vi "Main.vi"(8 "error in":errorcluster, 11 "Settings View in":refnum<class "Settings View.lvclass">) -> (0 "error out":errorcluster, 3 "Settings View out":refnum<class "Settings View.lvclass">)   [LabVIEW 2018, in "Settings View.lvclass"]
doc: "The Queued Message Handler of a Worker."
uses:
  Settings View.lvclass
  D:/Program Files (x86)/National Instruments/LabVIEW 2018/vi.lib/addons/_Workers/Library/Classes/Worker/Worker.lvclass
  Initialization Data.ctl
  Settings View.lvclass/Settings View.ctl
  <vilib>/addons/_Workers/Library/Classes/Worker/Worker.lvclass
panel:
  in  "TempSensor":refnum<visa-resource-name>
  in  "PS10":refnum<visa-resource-name>
  in  "PS9":refnum<visa-resource-name>
  in  "PS8":refnum<visa-resource-name>
  in  "PS7":refnum<visa-resource-name>
  in  "PS6":refnum<visa-resource-name>
  in  "PS5":refnum<visa-resource-name>
  in  "PS4":refnum<visa-resource-name>
  in  "PS3":refnum<visa-resource-name>
  in  "PS2":refnum<visa-resource-name>
  in  "PS1":refnum<visa-resource-name>
  in  "Save Button":bool
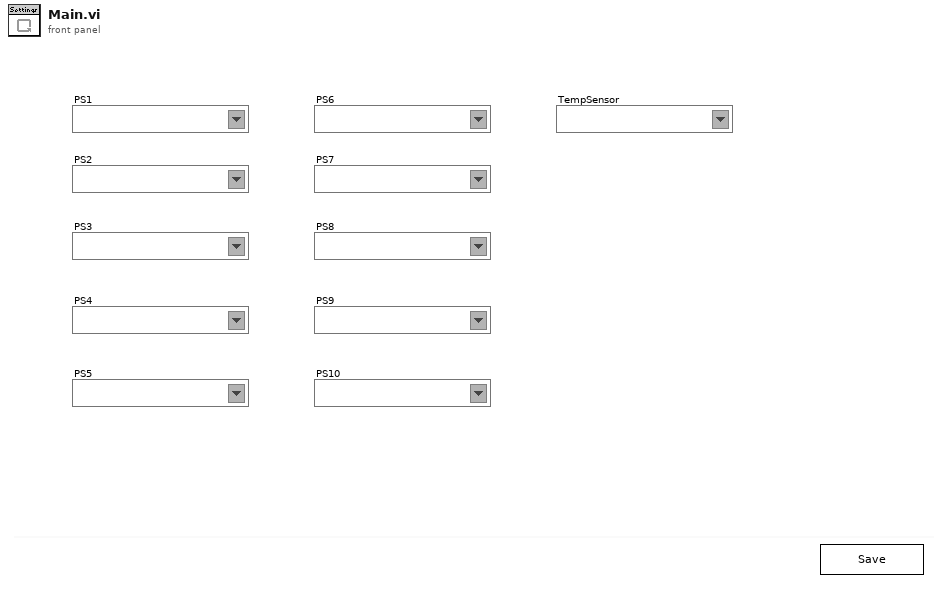
[diagram p1: front panel]
types:
  T1 = typedef "Settings View.lvclass/Initialization Data.ctl" = cluster{"MainPanel":refnum<vi>}
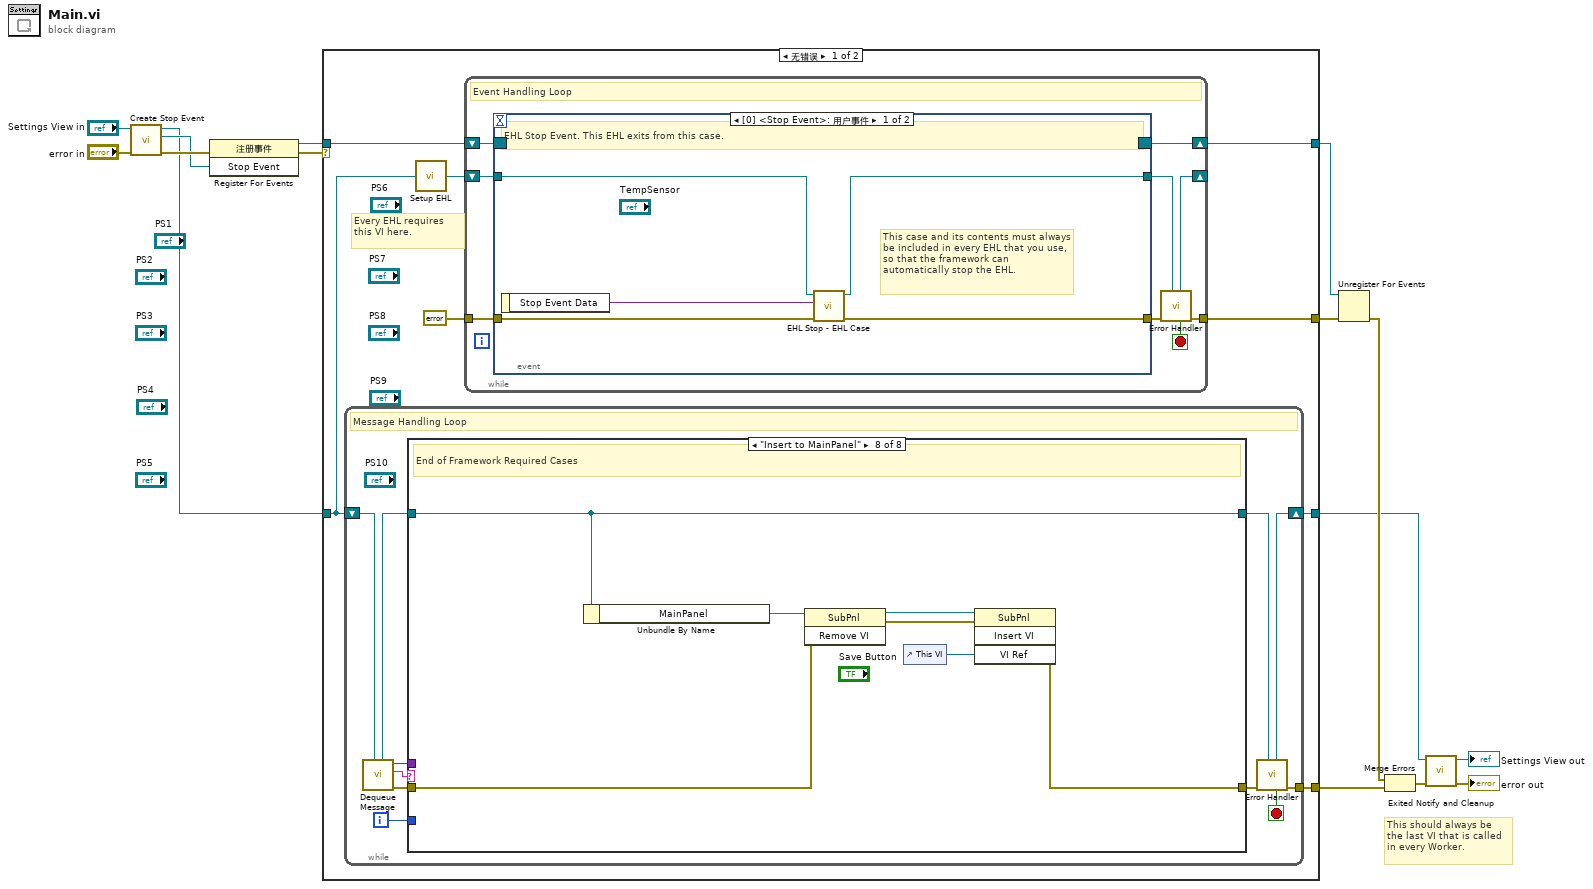
[diagram p0: block diagram]
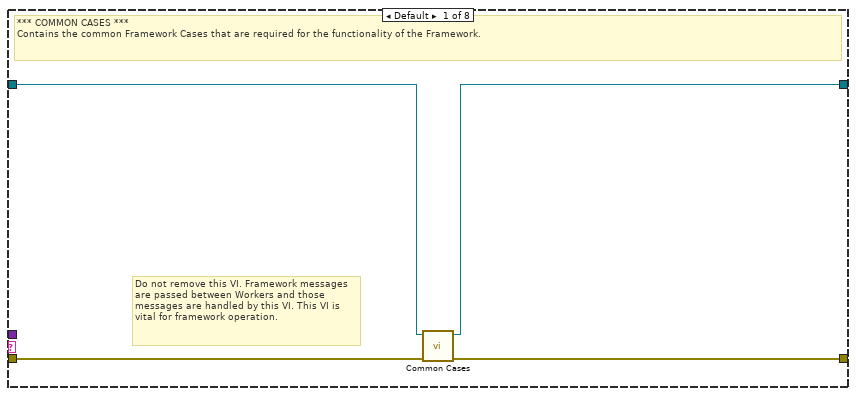
[diagram p2: hidden frame]
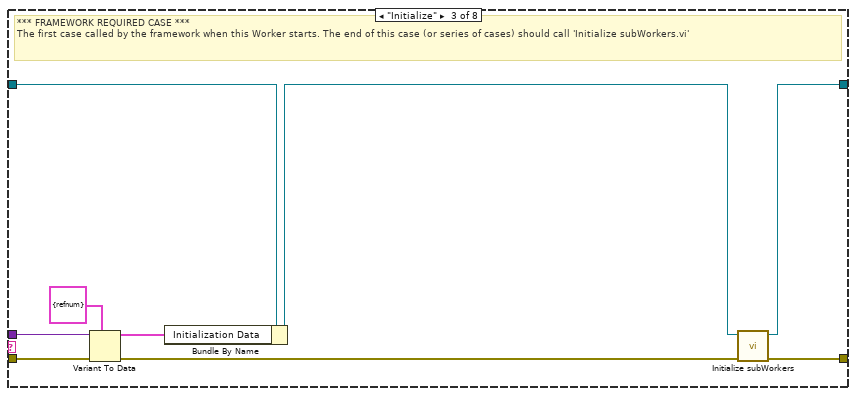
[diagram p4: hidden frame]
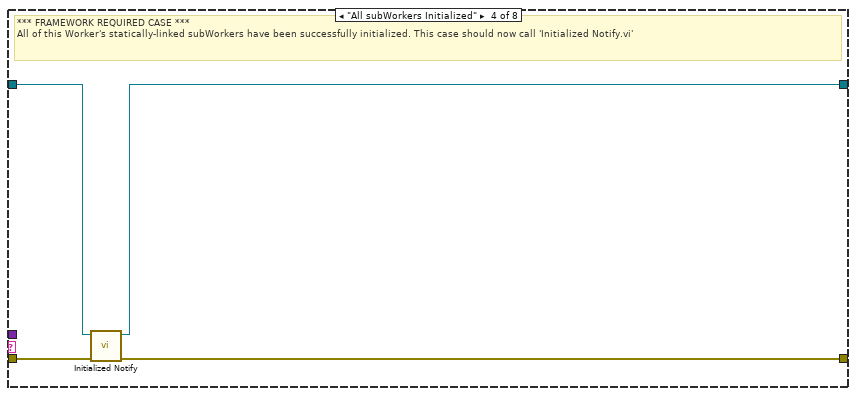
[diagram p5: hidden frame]
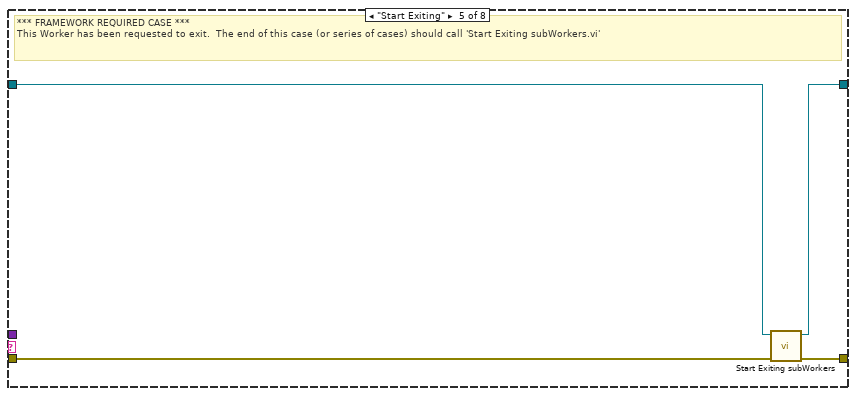
[diagram p6: hidden frame]
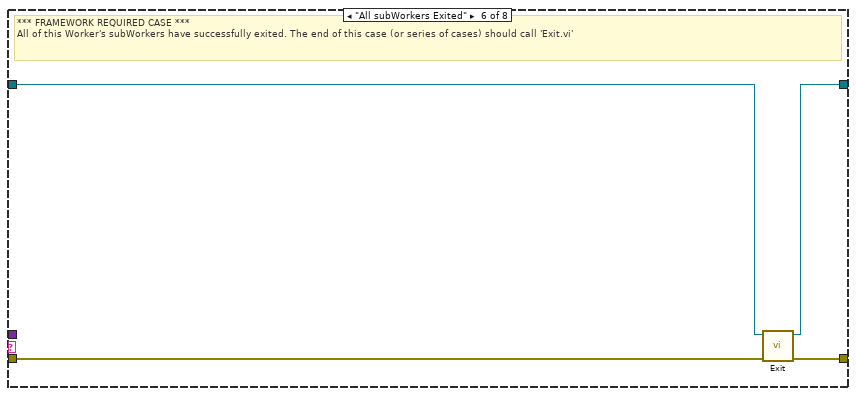
[diagram p7: hidden frame]
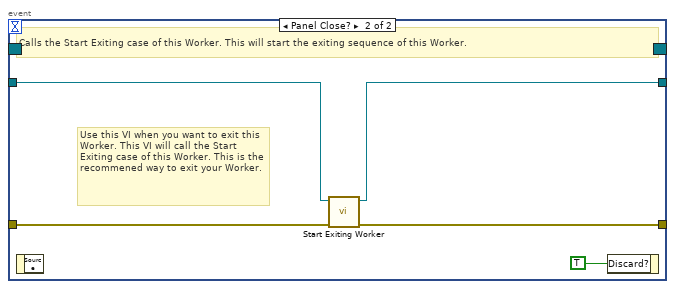
[diagram p9: hidden frame]
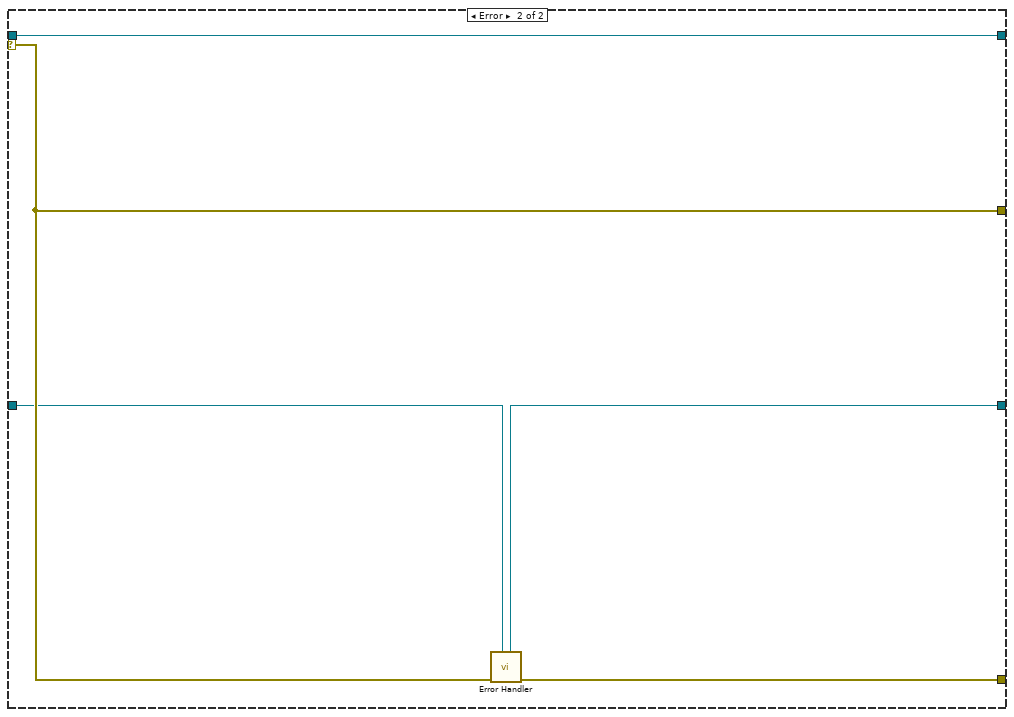
[diagram p10: hidden frame]
diagram:
  # "This should always be the last VI that is called in every Worker."
  n1 = call-dynamic "Create Stop Event.vi"("error in"="error in", "Worker"="Settings View in") -> ("error out"=w10:errorcluster, "Stop Event"=w7:refnum<user-event>, "Worker out"=w4:refnum<class "Settings View.lvclass">)  [unwired: 7 in]
  n2 = register-events(error in=w10, w7) -> (reference out=w9:refnum<event-registration>, error out=w1:errorcluster)  [unwired: 1 in]
  n3 = case shown="无错误" w1 {
    tunnel: w4 -> [w18 w91]
    tunnel: [w16 w92] -> w8
    tunnel: w9 -> [w23 w93]
    tunnel: [w20 w94] -> w14
    tunnel: [w22 w93] -> w13
    tunnel: [w17 w90] -> w11
    selector: w1 -> [_ w94]
    frame No Error {
      # "Every EHL requires\nthis VI here."
      n4 = while {
        shift-right: [w32] -> w17
        shift-left: w18 -> [w34]
        tunnel: [w33] -> w16
        i -> [w24]
        stop <- w25 stop-if-true
        # "Message Handling Loop"
        n5 = call-dynamic "Dequeue Message.vi"("Worker"=w34) -> ("error out"=w31:errorcluster, "Case out"=w26:string, "Data out"=w27:variant, "Worker out"=w29:refnum<class "Settings View.lvclass">)  [unwired: 6 in, 1 out]
        n6 = case "Worker MHL Case Structure (DO NOT CHANGE LABEL NAME)" shown="\"Insert to MainPanel\"" w26 {
          tunnel: w31 -> [w38 w39 w47 w51 w54 w61 w62 w65]
          tunnel: [w37 w39 w49 w50 w57 w60 w62 w64] -> w30
          tunnel: w29 -> [w36 w40 w46 w53 w55 w59 w63 w66]
          tunnel: [w35 w40 w48 w52 w56 w58 w63 w66] -> w28
          tunnel: w27 -> [_ _ w44 _ _ _ _ _]
          tunnel: w24 -> [_ _ _ _ _ _ _ _]
          frame Default {
            # "Do not remove this VI. Framework messages are passed between Workers and those messages are handled by this VI. This VI is vital for framework operation."
            # "*** COMMON CASES ***\nContains the common Framework Cases that are required for the functionality of the Framework."
            n7 = call-dynamic "Common Cases.vi"("error in"=w38, "Worker in"=w36) -> ("error out"=w37:errorcluster, "Worker out"=w35:refnum<class "Settings View.lvclass">)  [unwired: 8 in]
          }
          frame "------ FRAMEWORK REQUIRED CASES ------" {
            # "Start of Framework Required Cases"
          }
          frame "Initialize" {
            # "*** FRAMEWORK REQUIRED CASE ***\nThe first case called by the framework when this Worker starts. The end of this case (or series of cases) should call 'Initialize subWorkers.vi'"
            n8 = Variant To Data(error in=w47, type=T1 {"MainPanel"=refnum} ("Initialization Data"), Variant=w44) -> (data=w41:T1, error out=w45:errorcluster)
            n9 = Bundle By Name(cluster=w46, "Initialization Data"=w41) -> (w42:refnum<class "Settings View.lvclass">)
            n10 = call-dynamic "Initialize subWorkers.vi"("error in"=w45, "Worker"=w42) -> ("error out"=w49:errorcluster, "dup Worker out"=w48:refnum<class "Settings View.lvclass">)  [unwired: 8 in]
          }
          frame "All subWorkers Initialized" {
            # "*** FRAMEWORK REQUIRED CASE ***\nAll of this Worker's statically-linked subWorkers have been successfully initialized. This case should now call 'Initialized Notify.vi'"
            n11 = call-dynamic "Initialized Notify.vi"("error in"=w51, "Worker"=w53) -> ("error out"=w50:errorcluster, "dup Worker out"=w52:refnum<class "Settings View.lvclass">)  [unwired: 8 in]
          }
          frame "Start Exiting" {
            # "*** FRAMEWORK REQUIRED CASE ***\nThis Worker has been requested to exit.  The end of this case (or series of cases) should call 'Start Exiting subWorkers.vi'"
            n12 = call-dynamic "Start Exiting subWorkers.vi"("error_in"=w54, "Worker"=w55) -> ("error out"=w57:errorcluster, "dup Worker out"=w56:refnum<class "Settings View.lvclass">)  [unwired: 8 in]
          }
          frame "All subWorkers Exited" {
            # "*** FRAMEWORK REQUIRED CASE ***\nAll of this Worker's subWorkers have successfully exited. The end of this case (or series of cases) should call 'Exit.vi'"
            n13 = call-dynamic "Exit.vi"("error_in"=w61, "Worker"=w59) -> ("error out"=w60:errorcluster, "dup Worker out"=w58:refnum<class "Settings View.lvclass">)  [unwired: 8 in]
          }
          frame "-----------------------------------------------" {
            # "End of Framework Required Cases"
          }
          frame "Insert to MainPanel" {
            # "End of Framework Required Cases"
            n14 = Unbundle By Name(w66) -> ("MainPanel"=w70:refnum<vi>)
            n15 = invoke class="SubPnl" method="Remove VI"(reference=w70, error in=w65) -> (reference out=w69:refnum<vi>, error out=w68:errorcluster)  [unwired: 1 in, 1 out]
            n16 = control-ref of="This VI"() -> (w67:refnum<vi>)
            n17 = invoke class="SubPnl" method="Insert VI"(reference=w69, error in=w68, "VI Ref"=w67) -> (error out=w64:errorcluster)  [unwired: 1 in, 3 out]
          }
        }
        n18 = call-dynamic "Error Handler.vi"("Worker"=w28, "error_in"=w30) -> ("error out"=w33:errorcluster, "Stop Loop"=w25:bool, "Worker out"=w32:refnum<class "Settings View.lvclass">)  [unwired: 7 in]
      }
      n19 = call-dynamic "Setup EHL.vi"("Worker"=w18) -> ("Worker out"=w19:refnum<class "Settings View.lvclass">)  [unwired: 14 in]
      n20 = while "Event Handling Loop" {
        shift-right: [w79] -> w22
        shift-left: w23 -> [w78]
        tunnel: [w74] -> w20
        tunnel: errorcluster {"status"=FALSE, "code"=0, "source"=""} ("error constant") -> [w76]
        shift-right: [w72] -> _
        shift-left: w19 -> [w77]
        stop <- w71 stop-if-true
        # "Event Handling Loop"
        n21 = event shown="[0] <Stop Event>: 用户事件" {
          selector: w78 -> [_ _]
          dyn-events: [_ _] -> w79
          timeout: _ -> [_ _]
          tunnel: [w83 w88] -> w75
          tunnel: w76 -> [w84 w87]
          tunnel: w77 -> [w82 w86]
          tunnel: [w81 w85] -> w73
          event User Event {
            # "This case and its contents must always be included in every EHL that you use, so that the framework can automatically stop the EHL."
            # "EHL Stop Event. This EHL exits from this case."
            n22 = event-data() -> ("Stop Event Data"=w80:variant)  [unwired: 1 in]
            n23 = call <vilib>:"EHL Stop - EHL Case.vi"("error in"=w84, "Stop Event Data"=w80, "Worker"=w82) -> ("error out"=w83:errorcluster, "Worker out"=w81:refnum<class "Settings View.lvclass">)  [unwired: 7 in]
          }
          event Panel Close? {
            # "Use this VI when you want to exit this Worker. This VI will call the Start Exiting case of this Worker. This is the recommened way to exit your Worker."
            # "Calls the Start Exiting case of this Worker. This will start the exiting sequence of this Worker."
            n24 = event-data() -> ()  [unwired: 1 in, 1 out]
            n25 = call-dynamic "Start Exiting Worker.vi"("error in"=w87, "Worker"=w86) -> ("error out"=w88:errorcluster, "dup Worker out"=w85:refnum<class "Settings View.lvclass">)  [unwired: 8 in]
            n26 = event-data("Discard?"=TRUE) -> ()  [unwired: 1 in, 1 out]
          }
        }
        n27 = call-dynamic "Error Handler.vi"("Worker"=w73, "error_in"=w75) -> ("error out"=w74:errorcluster, "Stop Loop"=w71:bool, "Worker out"=w72:refnum<class "Settings View.lvclass">)  [unwired: 7 in]
      }
    }
    frame Error {
      n28 = call-dynamic "Error Handler.vi"("Worker"=w91, "error_in"=w94) -> ("error out"=w92:errorcluster, "Worker out"=w90:refnum<class "Settings View.lvclass">)  [unwired: 7 in, 1 out]
    }
  }
  n29 = Unregister For Events(event registration refnum=w13, error in=w14) -> (error out=w15:errorcluster)
  n30 = Merge Errors(w15, w8) -> (w12:errorcluster)
  n31 = call-dynamic "Exited Notify and Cleanup.vi"("error_in"=w12, "Worker"=w11) -> ("error out"=→"error out":errorcluster, "dup Worker out"=→"Settings View out":refnum<class "Settings View.lvclass">)  [unwired: 8 in]
